vi "Obtain Dense Array from Skeleton.vi"() -> ()   [LabVIEW 2016]
panel:
  in  "dB":dbl=0.1
  in  "Bf":dbl=9.0
  in  "B0":dbl
  out "Dense":cluster{dbl[], dbl[]}[](graph)=[{[0.0, 0.1, 0.2, 0.30000000000000004, 0.4, 0.5, 0.6000000000000001, 0.7000000000000001, 0.8, 0.9, 1.0, 1.1, 1.2000000000000002, 1.3, 1.4000000000000001, 1.5, 1.6, 1.7000000000000002, 1.8, 1.9000000000000001, 2.0, 2.1, 2.2, 2.3000000000000003, 2.4000000000000004, 2.5, 2.6, 2.7, 2.8000000000000003, 2.9000000000000004, 3.0, 3.1, 3.2, 3.3000000000000003, 3.4000000000000004, 3.5, 3.6, 3.7, 3.8000000000000003, 3.9000000000000004, 4.0, 4.1000000000000005, 4.2, 4.3, 4.4, 4.5, 4.6000000000000005, 4.7, 4.800000000000001, 4.9, 5.0, 5.1000000000000005, 5.2, 5.300000000000001, 5.4, 5.5, 5.6000000000000005, 5.7, 5.800000000000001, 5.9, 6.0, 6.1000000000000005, 6.2, 6.300000000000001, 6.4, 6.5, 6.6000000000000005, 6.7, 6.800000000000001, 6.9, 7.0, 7.1000000000000005, 7.2, 7.300000000000001, 7.4, 7.5, 7.6000000000000005, 7.7, 7.800000000000001, 7.9, 8.0, 8.1, 8.200000000000001, 8.3, 8.4, 8.5, 8.6, 8.700000000000001, 8.8, 8.9], [0.1702200000000002, 0.173952507868904, 0.17768501573780784, 0.18141752360671165, 0.18515003147561546, 0.1888825393445193, 0.1926150472134231, 0.1963475550823269, 0.20008006295123074, 0.20381257082013454, 0.20754507868903835, 0.21127758655794215, 0.215010094426846, 0.2187426022957498, 0.22247511016465363, 0.22620761803355743, 0.22994012590246124, 0.23367263377136505, 0.23740514164026888, 0.2411376495091727, 0.2448701573780765, 0.24860266524698033, 0.25233517311588416, 0.25606768098478794, 0.25980018885369177, 0.2635326967225956, 0.2672652045914994, 0.2709977124604032, 0.27473022032930705, 0.27846272819821083, 0.28219523606711466, 0.2859277439360185, 0.2896602518049223, 0.2933927596738261, 0.29712526754272994, 0.3008577754116337, 0.30459028328053755, 0.3083227911494414, 0.31205529901834517, 0.315787806887249, 0.31952031475615283, 0.3232528226250566, 0.32698533049396045, 0.3307178383628643, 0.33445034623176806, 0.33818285410067184, 0.3419153619695757, 0.3456478698384795, 0.3493803777073834, 0.35311288557628717, 0.35684539344519095, 0.36057790131409484, 0.3643104091829986, 0.3680429170519024, 0.37177542492080623, 0.37550793278971006, 0.37924044065861384, 0.3829729485275177, 0.3867054563964215, 0.3904379642653253, 0.39417047213422907, 0.39790298000313296, 0.40163548787203673, 0.4053679957409406, 0.4091005036098444, 0.4128330114787482, 0.416565519347652, 0.4202980272165558, 0.4235448227695398, 0.42564606461511, 0.42774730646068027, 0.42984854830625047, 0.43194979015182067, 0.4340510319973909, 0.43709182498285537, 0.44140769268401087, 0.4457235603851664, 0.4500394280863219, 0.4543552957874774, 0.4586711634886329, 0.4629870311897884, 0.4673028988909439, 0.47161876659209945, 0.475934634293255, 0.4802505019944105, 0.48456636969556593, 0.48888223739672143, 0.49319810509787704, 0.49751397279903253, 0.501829840500188]}, {[0.0, 0.1, 0.2, 0.30000000000000004, 0.4, 0.5, 0.6000000000000001, 0.7000000000000001, 0.8, 0.9, 1.0, 1.1, 1.2000000000000002, 1.3, 1.4000000000000001, 1.5, 1.6, 1.7000000000000002, 1.8, 1.9000000000000001, 2.0, 2.1, 2.2, 2.3000000000000003, 2.4000000000000004, 2.5, 2.6, 2.7, 2.8000000000000003, 2.9000000000000004, 3.0, 3.1, 3.2, 3.3000000000000003, 3.4000000000000004, 3.5, 3.6, 3.7, 3.8000000000000003, 3.9000000000000004, 4.0, 4.1000000000000005, 4.2, 4.3, 4.4, 4.5, 4.6000000000000005, 4.7, 4.800000000000001, 4.9, 5.0, 5.1000000000000005, 5.2, 5.300000000000001, 5.4, 5.5, 5.6000000000000005, 5.7, 5.800000000000001, 5.9, 6.0, 6.1000000000000005, 6.2, 6.300000000000001, 6.4, 6.5, 6.6000000000000005, 6.7, 6.800000000000001, 6.9, 7.0, 7.1000000000000005, 7.2, 7.300000000000001, 7.4, 7.5, 7.6000000000000005, 7.7, 7.800000000000001, 7.9, 8.0, 8.1, 8.200000000000001, 8.3, 8.4, 8.5, 8.6, 8.700000000000001, 8.8, 8.9], [0.35151, 0.35256475336753057, 0.35361950673506115, 0.3546742601025918, 0.35572901347012237, 0.35678376683765295, 0.35783852020518353, 0.3588932735727141, 0.3599480269402447, 0.36100278030777533, 0.3620575336753059, 0.3631122870428365, 0.36416704041036707, 0.36522179377789765, 0.3662765471454283, 0.36733130051295887, 0.36838605388048945, 0.36944080724802003, 0.3704955606155506, 0.37155031398308125, 0.37260506735061183, 0.3736598207181424, 0.374714574085673, 0.37576932745320357, 0.37682408082073415, 0.3778788341882648, 0.37893358755579537, 0.37998834092332595, 0.38104309429085653, 0.3820978476583871, 0.3831526010259177, 0.38420735439344833, 0.3852621077609789, 0.3863168611285095, 0.3873716144960401, 0.38842636786357065, 0.38948112123110123, 0.39053587459863187, 0.39159062796616245, 0.39264538133369303, 0.3937001347012236, 0.39475488806875425, 0.39580964143628483, 0.3968643948038154, 0.397919148171346, 0.3989739015388766, 0.40002865490640716, 0.4010834082739378, 0.4021381616414684, 0.40319291500899895, 0.40424766837652953, 0.4053024217440601, 0.4063571751115907, 0.40741192847912133, 0.4084666818466519, 0.4095214352141825, 0.4105761885817131, 0.41163094194924366, 0.4126856953167743, 0.4137404486843049, 0.41479520205183545, 0.41584995541936604, 0.4169047087868966, 0.41795946215442725, 0.41901421552195783, 0.4200689688894884, 0.421123722257019, 0.4221784756245496, 0.4235448227695398, 0.42564606461511, 0.42774730646068027, 0.42984854830625047, 0.43194979015182067, 0.4340510319973909, 0.43554953374516947, 0.43623005057845593, 0.43691056741174245, 0.4375910842450289, 0.4382716010783154, 0.4389521179116019, 0.43963263474488834, 0.44031315157817486, 0.4409936684114613, 0.4416741852447478, 0.4423547020780343, 0.44303521891132075, 0.4437157357446072, 0.4443962525778937, 0.4450767694111802, 0.4457572862444667]}]
  in  "Skeleton":cluster{dbl[], dbl[]}[](graph)=[{[0.0, 6.7763179034335925, 7.312482096566412, 9.0], [0.17059000000000035, 0.4230678280216815, 0.43421217197831685, 0.5059196708591177]}, {[0.0, 6.7763179034335925, 7.312482096566412, 9.0], [0.35147, 0.4230678280216815, 0.43421217197831685, 0.44656300793999393]}]
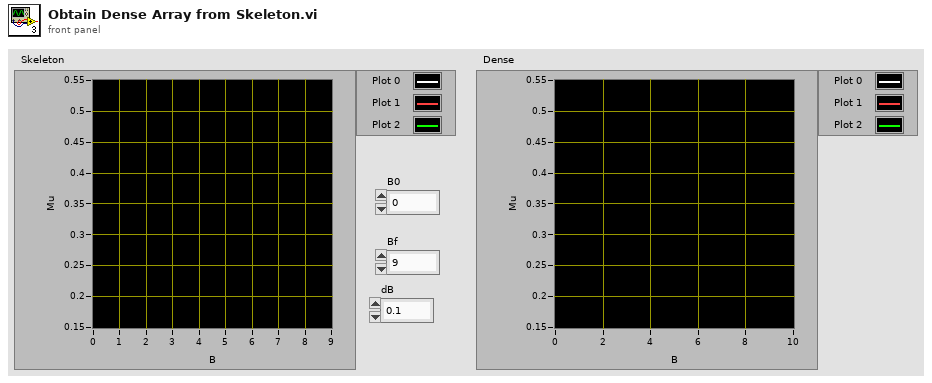
[diagram p1: front panel]
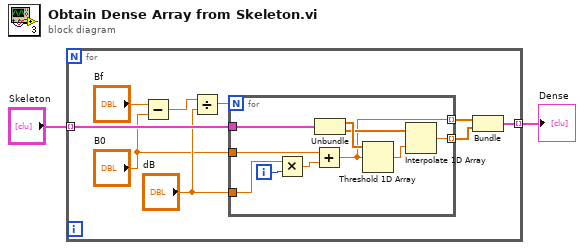
[diagram p0: block diagram]
diagram:
  n1 = for {
    tunnel: "Skeleton" -> [w11] mode=indexing
    tunnel: [w5] -> w1 mode=indexing
    n2 = Subtract(x="Bf", y="B0") -> (x-y=w9:dbl)
    n3 = Divide(x=w9, y="dB") -> (x/y=w8:dbl)
    n4 = for {
      N: w8 -> [_]
      tunnel: w11 -> [w21]
      tunnel: "dB" -> [w18]
      tunnel: [w14] -> w6 mode=indexing
      tunnel: [w12] -> w4 mode=indexing
      tunnel: "B0" -> [w13]
      i -> [w19]
      n5 = Multiply(x=w18, y=w19) -> (x*y=w20:dbl)
      n6 = Add(x=w13, y=w20) -> (x+y=w12:dbl)
      n7 = Unbundle(w21) -> (w17:dbl[], w15:dbl[])
      n8 = Threshold 1D Array(2:w12, 3:w17) -> (0:w16:dbl)  [unwired: 1 in]
      n9 = Interpolate 1D Array(1:w16, 2:w15) -> (0:w14:dbl)
    }
    n10 = Bundle(w4, w6) -> (w5:cluster{dbl[], dbl[]})  [unwired: 1 in]
  }
  "Dense" <- w1
